vi "get Remaining Idle Time.vi"(11 "Timer in":refnum<class "Timer.lvclass">) -> (3 "Remaining Idle Time [s]":dbl)   [LabVIEW 2015, in "Timer.lvclass"]
uses:
  Timer.lvclass
  Timer.lvclass/Timer.ctl
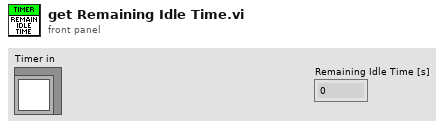
[diagram p1: front panel]
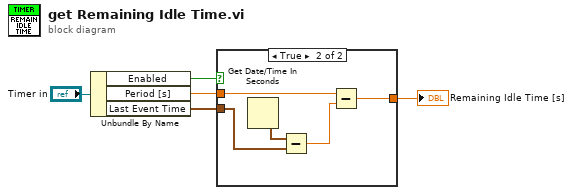
[diagram p0: block diagram]
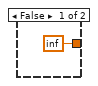
[diagram p2: hidden frame]
diagram:
  n1 = Unbundle By Name("Timer in") -> ("Enabled"=w1:bool, "Period [s]"=w2:dbl, "Last Event Time"=w3:timestamp)
  n2 = case shown="True" w1 {
    tunnel: w3 -> [_ w8]
    tunnel: w2 -> [_ w11]
    tunnel: [inf w10] -> w4
    frame False {
    }
    frame True {
      n3 = Get Date/Time In Seconds() -> (seconds since 1Jan1904=w9:timestamp)
      n4 = Subtract(x=w9, y=w8) -> (x-y=w7:dbl)
      n5 = Subtract(x=w11, y=w7) -> (x-y=w10:dbl)
    }
  }
  "Remaining Idle Time [s]" <- w4
